vi "Convert Move Command.vi"(8 "error in":errorcluster, 11 "Position in":i32[](array[numeric])) -> (0 "error out":errorcluster, 3 "Command out":string)   [LabVIEW 2019, in "Allmotion.lvlib"]
uses:
  Allmotion.lvlib
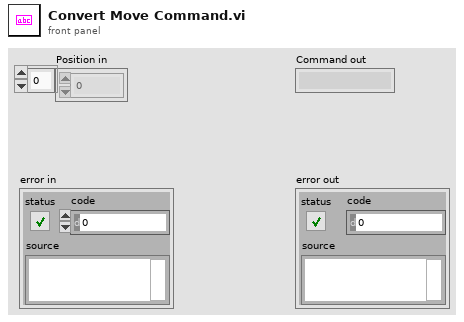
[diagram p1: front panel]
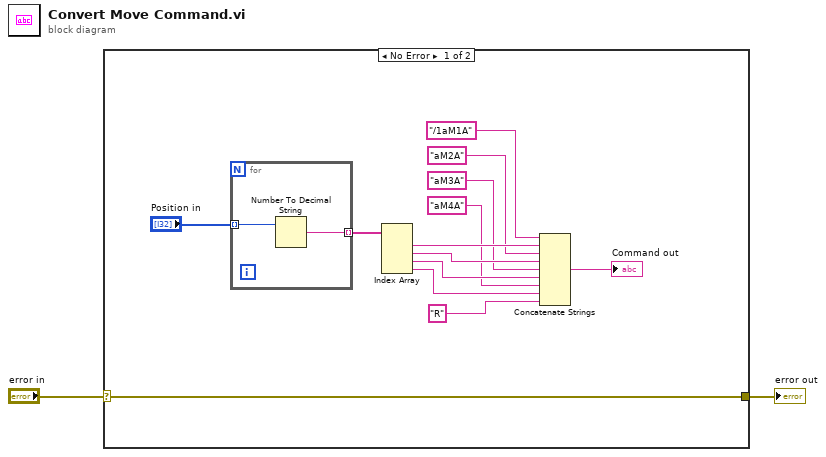
[diagram p0: block diagram]
diagram:
  n1 = case shown="No Error" "error in" {
    selector: "error in" -> [w3 w18]
    tunnel: [w3 w18] -> w1
    frame No Error {
      n2 = for {
        tunnel: "Position in" -> [w17] mode=indexing
        tunnel: [w16] -> w14 mode=indexing
        n3 = Number To Decimal String(number=w17) -> (decimal integer string=w16:string)  [unwired: 1 in]
      }
      n4 = Index Array(array=w14) -> (element #1=w12:string, element #2=w11:string, element #3=w10:string, element #4=w9:string)  [unwired: 4 in]
      n5 = Concatenate Strings("/1aM1A", w12, "aM2A", w11, "aM3A", w10, "aM4A", w9, "R") -> (→"Command out":string)
    }
    frame Error {
    }
  }
  "error out" <- w1
